vi "hmi_halo_drive.vi"(4 "QuickTurn Const":dbl=0.25, 6 "Turn Gains":T1={"Quickturn_Sens_Low"=1.2, "Quickturn_Sens_High"=1.0, "Speedturn_Sens_Low"=1.5, "Speedturn_Sens_High"=1.7}, 10 "Wheel":dbl, 11 "Throttle":dbl) -> (3 "Drive Data":cluster{"Left":dbl, "Right":dbl})   [LabVIEW 2013]
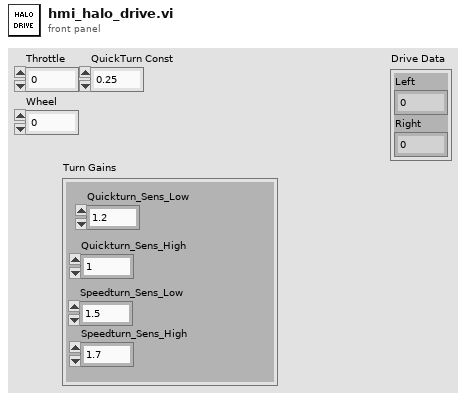
[diagram p1: front panel]
types:
  T1 = cluster{"Quickturn_Sens_Low":dbl, "Quickturn_Sens_High":dbl, "Speedturn_Sens_Low":dbl, "Speedturn_Sens_High":dbl}
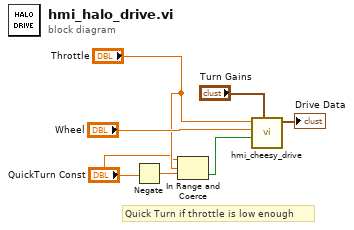
[diagram p0: block diagram]
diagram:
  # "Quick Turn if throttle is low enough"
  n1 = Negate(x="QuickTurn Const") -> (-x=w4:dbl)
  n2 = In Range and Coerce(upper limit="QuickTurn Const", x="Throttle", lower limit=w4) -> (In Range?=w2:bool)  [unwired: 1 out]
  n3 = call "hmi_cheesy_drive.vi"("Turn Gains"="Turn Gains", "Quick Turn"=w2, "Wheel"="Wheel", "Throttle"="Throttle") -> ("Drive Data"=→"Drive Data":cluster{"Left":dbl, "Right":dbl})  [unwired: 7 in]
